vi "Reemplace build.vi"(9 "index":i32, 10 "build modified":T1={"App Name"="", "Build Type"=enum."Fix", "Current Version"="", "Next Version"="", "Check"=FALSE}, 11 "Builder in":refnum<class "Builder.lvclass">) -> (3 "Builder out":refnum<class "Builder.lvclass">)   [LabVIEW 2021, in "App-Builder Library.lvlib" / "Builder.lvclass"]
uses:
  Builder.lvclass
  Build Type.ctl
  App descriptions.ctl
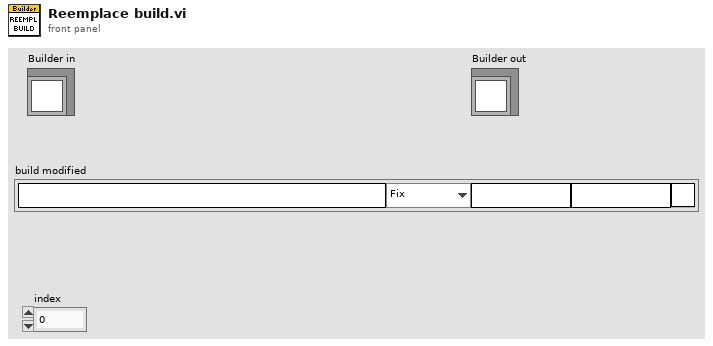
[diagram p1: front panel]
types:
  T1 = typedef "App-Builder Library.lvlib/Builder.lvclass/App descriptions.ctl" = cluster{"App Name":string, "Build Type":T2, "Current Version":string, "Next Version":string, "Check":bool}
  T2 = typedef "App-Builder Library.lvlib/Builder.lvclass/Build Type.ctl" = enum16{"Major", "Minor", "Fix", "Build"}
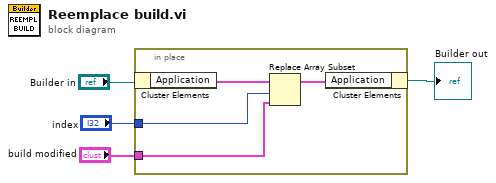
[diagram p0: block diagram]
diagram:
  n1 = in-place {
    in-place-border: "index" -> [w8]
    in-place-border: "build modified" -> [w7]
    n2 = in-place-cluster #1("Builder in") -> ("Application"=w6:T1[])
    n3 = Replace Array Subset(array=w6, new element=w7, index=w8) -> (w5:T1[])
    n4 = in-place-cluster #1("Application"=w5) -> (→"Builder out":refnum<class "Builder.lvclass">)
  }
